vi "Test unknown report file type.vi"(8 "error in (no error)":errorcluster, 11 "API Test in":refnum<class "API Test.lvclass">) -> (0 "error out":errorcluster, 3 "API Test out":refnum<class "API Test.lvclass">)   [LabVIEW 2020, in "LUnit Tests.lvlib" / "API Test.lvclass"]
uses:
  API Test.lvclass
  source/Framework/Execution API/Execution API.lvclass
  <vilib>/Astemes/LUnit/Test Case.lvclass
  C:/Program Files (x86)/National Instruments/LabVIEW 2020/vi.lib/Astemes/LUnit/Test Case.lvclass
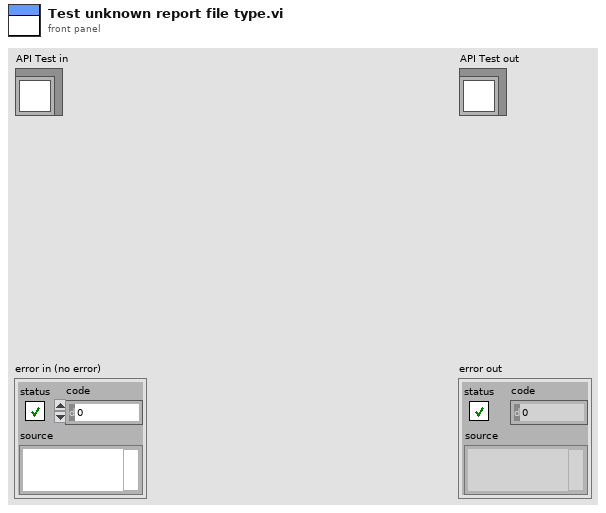
[diagram p1: front panel]
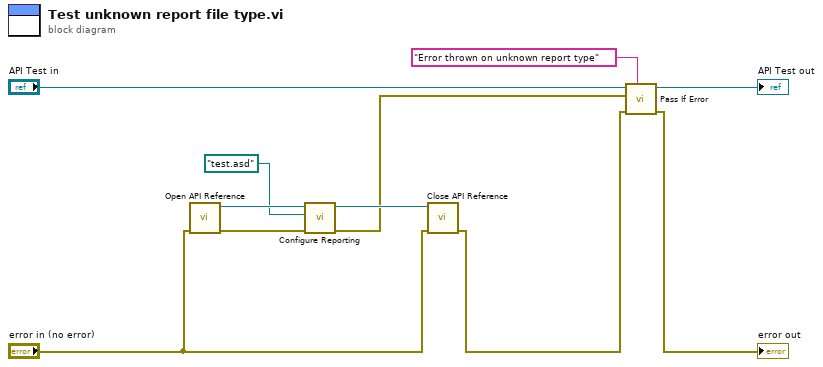
[diagram p0: block diagram]
diagram:
  n1 = call "Open API Reference.vi"("error in (no error)"="error in (no error)") -> ("error out"=w9:errorcluster, "Execution API out"=w10:refnum<class "Execution API.lvclass">)  [unwired: 9 in]
  n2 = call "Configure Reporting.vi"("error in (no error)"=w9, "Path"=path "test.asd", "Execution API In"=w10) -> ("error out"=w3:errorcluster, "Execution API Out"=w8:refnum<class "Execution API.lvclass">)  [unwired: 7 in]
  n3 = call "Close API Reference.vi"("error in (no error)"="error in (no error)", "Execution API in"=w8) -> ("error out"=w1:errorcluster)  [unwired: 9 in]
  n4 = call <vilib>:"Pass If Error.vi"("Description"="Error thrown on unknown report type", "error in (no error)"=w1, "Assert error"=w3, "LUnit Test Case In"="API Test in") -> ("error out"=→"error out":errorcluster, "LUnit Test Case Out"=→"API Test out":refnum<class "API Test.lvclass">)  [unwired: 6 in]
